vi "Set Bias Voltage.vi"(8 "error in (no error)":errorcluster, 9 "Channel":i32, 10 "Bias Voltage (V)":dbl, 11 "Example in":refnum<class "Instrument.FrameworkTemplate.lvclass">) -> (0 "error out":errorcluster, 3 "Example out":refnum<class "Instrument.FrameworkTemplate.lvclass">)   [LabVIEW 2019, in "Instrument.FrameworkTemplate.lvclass"]
uses:
  Instrument.FrameworkTemplate.lvclass
  C:/Program Files (x86)/National Instruments/LabVIEW 2019/user.lib/LevyLab/Instrument Framework/SMOs/Instrument/Instrument.lvclass
  Typedefs/Instrument.FrameworkTemplate.Commands--Enum.ctl
  <userlib>/LevyLab/Instrument Framework/SMOs/Instrument/Instrument.lvclass/Instrument.ctl
  67792bfe-8e2c-4879-abc2-cb448bcec168.vi
  67792bfe-8e2c-4879-abc2-cb448bcec168.vi/e8961c42-2f1b-4108-af53-b9099feb00cd.vi
  <userlib>/LevyLab/Instrument Framework/SMOs/Instrument/API/Send and Receive.vi
  67792bfe-8e2c-4879-abc2-cb448bcec168.vi/e8961c42-2f1b-4108-af53-b9099feb00cd.vi/7ce7854a-098b-4e2f-bcb9-3cabce4f14f9.vi
  67792bfe-8e2c-4879-abc2-cb448bcec168.vi/e8961c42-2f1b-4108-af53-b9099feb00cd.vi/5e1fe7a6-e2f1-46bf-8fd0-2fa8f727542d.vi
  <userlib>/LevyLab/Instrument Framework/SMOs/Instrument/API/Enum to String.vi
  <userlib>/LevyLab/Instrument Framework/SMOs/RemoteControl/API/Send and Receive.vi
  <vilib>/Utility/Data Type/Get Type Information.vi
  <vilib>/JDP Science/JSONtext/JSON text to Variant.vi
  <vilib>/JDP Science/JSONtext/LVClass Serializer/JSONtext LVClass Serializer.lvclass
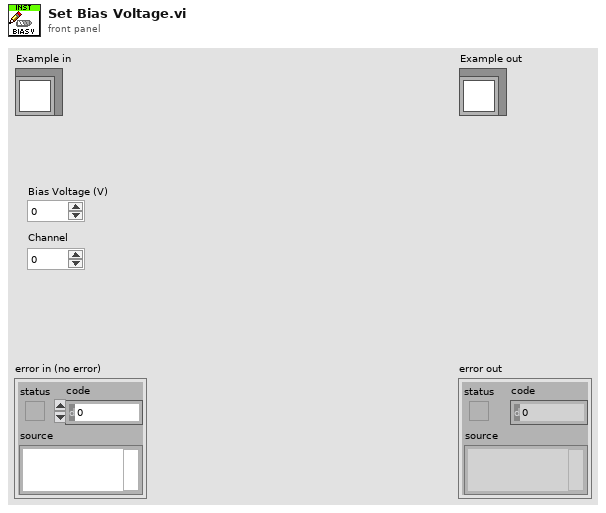
[diagram p1: front panel]
types:
  T1 = typedef "Instrument.FrameworkTemplate.lvclass/Instrument.FrameworkTemplate.Commands--Enum.ctl" = enum16{"command0", "command1", "command2"}
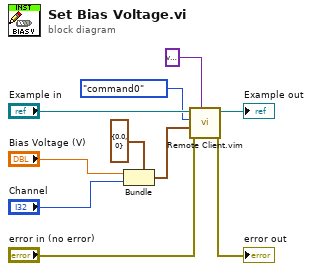
[diagram p0: block diagram]
diagram:
  n1 = Bundle(cluster=cluster{"Bias Voltage (V)":dbl, "Channel":i32} {"Bias Voltage (V)"=0.0, "Channel"=0} ("output cluster"), "Bias Voltage (V)"="Bias Voltage (V)", "Channel"="Channel") -> (w3:cluster{"Bias Voltage (V)":dbl, "Channel":i32})
  n2 = call "Remote Client.vim"("Data Out type"=variant, "error in (no error)"="error in (no error)", "params"=w3, "method"=Instrument.FrameworkTemplate.Commands--Enum."command0" ("Commands"), "Instrument in"="Example in") -> ("error out"=→"error out":errorcluster, "Instrument out"=→"Example out":refnum<class "Instrument.FrameworkTemplate.lvclass">)  [unwired: 3 in, 2 out]
